vi "Move single motor.vi"(6 "Avance":dbl=1.0 format="%#_g°", 7 "Position in":cluster{"M1 pos":dbl, "M2 pos ":dbl}, 8 "error in (no error)":errorcluster, 10 "Motor params":T4, 11 "DAQ Module ID":i32) -> (0 "error out":errorcluster, 2 "WHL args":T2)   [LabVIEW 2020]
uses:
  controls/Motor direction ---typedef.ctl
  Controls/Motor controls---typedef.ctl
  controls/Continuous acquisition ---argument.ctl
  controls/Motor FGV states ---typedef.ctl
  controls/Motor params ---typedef.ctl
panel:
  out "Motor control out":T1
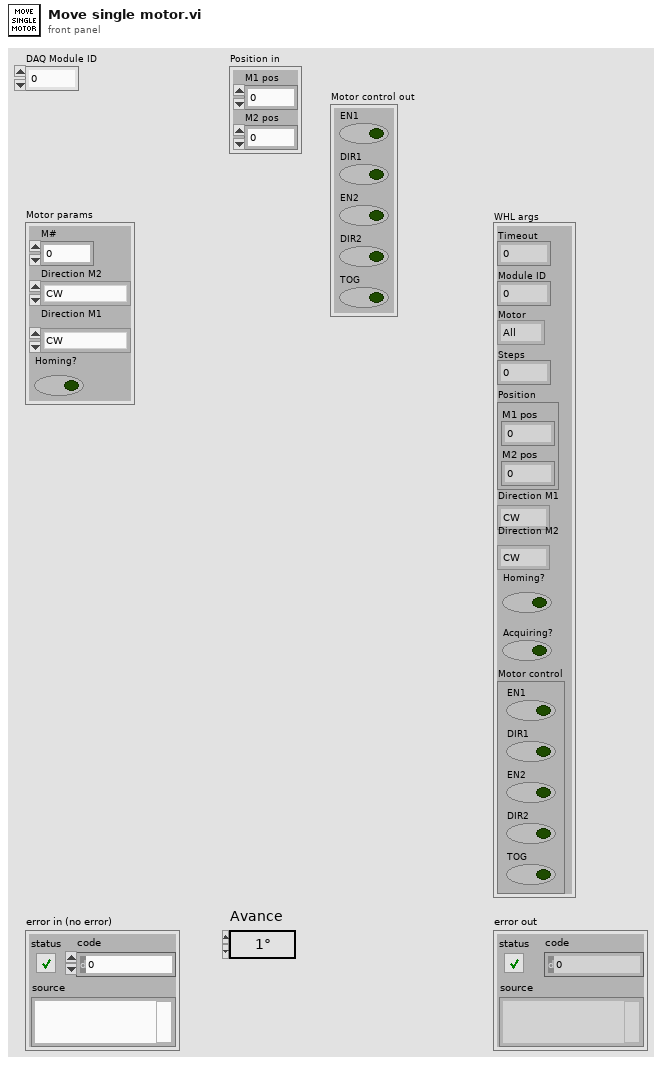
[diagram p1: front panel]
types:
  T1 = typedef "Motor controls---typedef.ctl" = cluster{"EN1":bool, "DIR1":bool, "EN2":bool, "DIR2":bool, "TOG":bool}
  T2 = typedef "Continuous acquisition ---argument.ctl" = cluster{"Timeout":i32, "Module ID":i32, "Motor":enum16{"All", "M1", "M2"}, "Steps":i32, "Position":cluster{"M1 pos":dbl, "M2 pos ":dbl}, "Direction M1":T3, "Direction M2":T3, "Homing?":bool, "Acquiring?":bool, "Motor control":T1}
  T3 = typedef "Motor direction ---typedef.ctl" = enum16{"CW", "CCW"}
  T4 = typedef "Motor params ---typedef.ctl" = cluster{"M#":i32, "Direction M2":T3, "Direction M1":T3, "Homing?":bool}
  T5 = typedef "Motor FGV states ---typedef.ctl" = enum16{"Set", "Reset", "Get"}
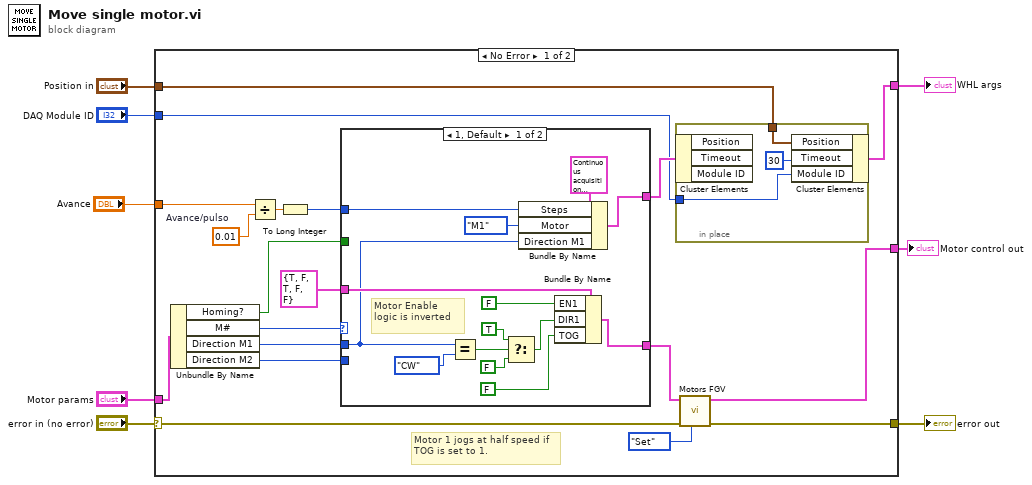
[diagram p0: block diagram]
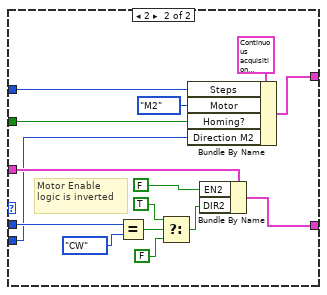
[diagram p2: hidden frame]
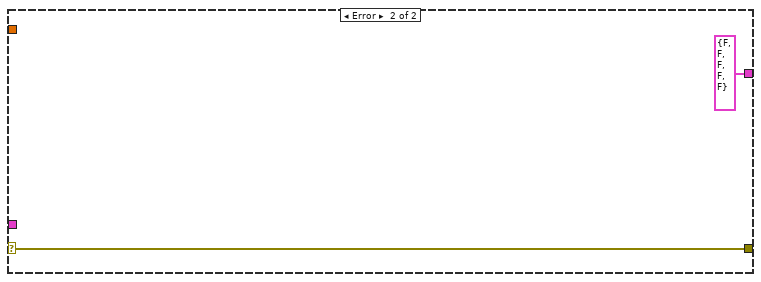
[diagram p3: hidden frame]
diagram:
  n1 = case shown="No Error" "error in (no error)" {
    selector: "error in (no error)" -> [w17 w61]
    tunnel: [w12 w61] -> w8
    tunnel: "DAQ Module ID" -> [w11 _]
    tunnel: "Motor params" -> [w24 _]
    tunnel: "Avance" -> [w23 _]
    tunnel: [w19 _] -> w3
    tunnel: "Position in" -> [w18 _]
    tunnel: [w10 T1 {"EN1"=FALSE, "DIR1"=FALSE, "EN2"=FALSE, "DIR2"=FALSE, "TOG"=FALSE} ("Motor control out")] -> w1
    frame No Error {
      w22 = 0.01  # Avance/pulso
      # "Motor 1 jogs at half speed if TOG is set to 1."
      n2 = Unbundle By Name(w24) -> ("Homing?"=w13:bool, "M#"=w25:i32, "Direction M1"=w27:T3, "Direction M2"=w9:T3)
      n3 = Divide(x=w23, y=w22) -> (x/y=w21:dbl)
      n4 = To Long Integer(number=w21) -> (32bit integer=w20:i32)
      n5 = case shown="1, Default" w25 {
        tunnel: T1 {"EN1"=TRUE, "DIR1"=FALSE, "EN2"=TRUE, "DIR2"=FALSE, "TOG"=FALSE} ("Motor control") -> [w44 w59]
        tunnel: w27 -> [w32 w47]
        tunnel: w20 -> [w35 w50]
        tunnel: [w34 w51] -> w16
        tunnel: [w31 w48] -> w15
        tunnel: w13 -> [_ w46]
        tunnel: w9 -> [_ w45]
        frame 1, Default {
          # "Motor Enable logic is inverted"
          n6 = Equal?(x=w32, y=Motor_direction_---typedef."CW") -> (x = y?=w41:bool)
          n7 = Select(t=TRUE ("EN1"), s=w41, f=FALSE) -> (s? t:f=w38:bool)
          n8 = Bundle By Name(cluster=T2 {"Timeout"=0, "Module ID"=0, "Motor"=enum."All", "Steps"=0, "Position"={"M1 pos"=0.0, "M2 pos "=0.0}, "Direction M1"=enum."CW", "Direction M2"=enum."CW", "Homing?"=FALSE, "Acquiring?"=FALSE, "Motor control"={"EN1"=FALSE, "DIR1"=FALSE, "EN2"=FALSE, "DIR2"=FALSE, "TOG"=FALSE}} ("event data"), "Steps"=w35, "Motor"=enum16{"All", "M1", "M2"}."M1", "Direction M1"=w32) -> (w34:T2)
          n9 = Bundle By Name(cluster=w44, "EN1"=FALSE, "DIR1"=w38, "TOG"=FALSE) -> (w31:T1)
        }
        frame 2 {
          # "Motor Enable logic is inverted"
          n10 = Equal?(x=w47, y=Motor_direction_---typedef."CW") -> (x = y?=w56:bool)
          n11 = Select(t=TRUE ("EN1"), s=w56, f=FALSE) -> (s? t:f=w53:bool)
          n12 = Bundle By Name(cluster=T2 {"Timeout"=0, "Module ID"=0, "Motor"=enum."All", "Steps"=0, "Position"={"M1 pos"=0.0, "M2 pos "=0.0}, "Direction M1"=enum."CW", "Direction M2"=enum."CW", "Homing?"=FALSE, "Acquiring?"=FALSE, "Motor control"={"EN1"=FALSE, "DIR1"=FALSE, "EN2"=FALSE, "DIR2"=FALSE, "TOG"=FALSE}} ("event data"), "Steps"=w50, "Motor"=enum16{"All", "M1", "M2"}."M2", "Homing?"=w46, "Direction M2"=w45) -> (w51:T2)
          n13 = Bundle By Name(cluster=w59, "EN2"=FALSE ("EN1"), "DIR2"=w53) -> (w48:T1)
        }
      }
      n14 = in-place {
        in-place-border: w11 -> [w29]
        in-place-border: w18 -> [w28]
        n15 = in-place-cluster #1(w16) -> ()  [unwired: 3 out]
        n16 = in-place-cluster #1("Position"=w28, "Timeout"=30, "Module ID"=w29) -> (w19:T2)
      }
      n17 = call "Motors FGV.vi"("Action"=Motor_FGV_states_---typedef."Set", "error in (no error)"=w17, "Motor control in"=w15) -> ("error out"=w12:errorcluster, "Motor control out"=w10:T1)  [unwired: 7 in]
    }
    frame Error {
    }
  }
  "error out" <- w8
  "WHL args" <- w3
  "Motor control out" <- w1
